vi "Configure DRAM Properties.vi"(7 "DRAM FIFO Depth":u8(ring)=20 items=["4"=2, "8"=3, "16"=4, "32"=5, "64"=6, "128"=7, "256"=8, "512"=9, "1024"=10, "2048"=11, "4096"=12, "8192"=13, "16384"=14, "32768"=15, "65536"=16, "131072"=17, "262144"=18, "524288"=19, "1048576"=20, "2097152"=21, "4194304"=22, "8388608"=23, "16777216"=24, "33554432"=25, "67108864"=26, "134217728"=27, "268435456"=28, "536870912"=29, "1073741824"=30, "2147483648"=31, "4294967296"=32], 8 "error in":errorcluster, 9 "DRAM Duty Cycle":T1={"DRAM Write Ticks"=1000, "DRAM Read Ticks"=1}, 11 "FPGA VI Reference In":refnum<k20>) -> (0 "error out":errorcluster, 3 "FPGA VI Reference Out":refnum<k20>)   [LabVIEW 2012]
uses:
  <vilib>/Utility/error.llb/Error Cluster From Error Code.vi
  <vilib>/rvi/errors/niLvFpgaAdjustHostInterfaceError.vi
  <vilib>/rvi/interface/nirviReadWriteControl/nirviReadWriteControl.xnode
  NiFpgaLv.dll
  <vilib>/rvi/interface/Simulation/niFpgaSimulationCallBeginRW.vi
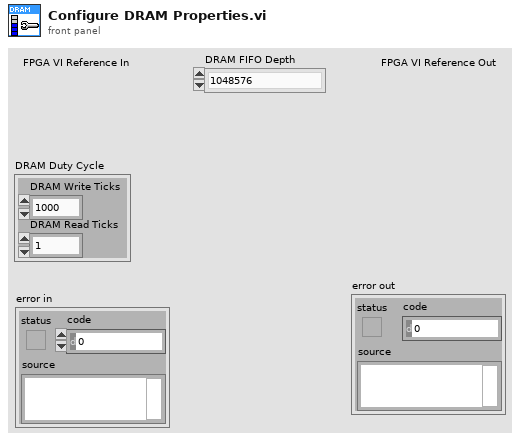
[diagram p1: front panel]
types:
  T1 = cluster{"DRAM Write Ticks":u16, "DRAM Read Ticks":u16}
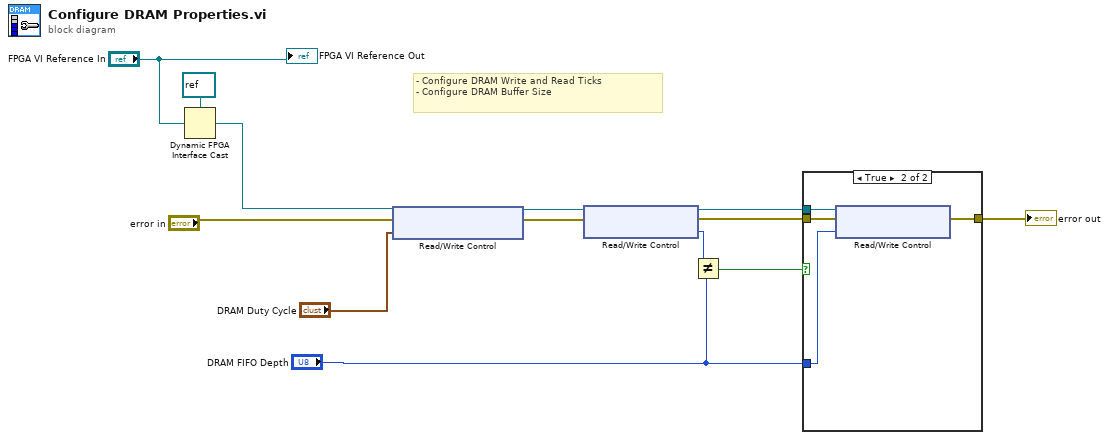
[diagram p0: block diagram]
diagram:
  # "- Configure DRAM Write and Read Ticks\n- Configure DRAM Buffer Size"
  n1 = Dynamic FPGA Interface Cast(Session In=refnum<k20> refnum ("Type"), Type="FPGA VI Reference In") -> (Session Out=w11:refnum<k20>)
  n2 = xnode "Read/Write Control"("FPGA VI Reference In"=w11, "error in"="error in", "DRAM Arbiter Config"="DRAM Duty Cycle") -> ("FPGA VI Reference Out"=w7:refnum<k20>, "error out"=w6:errorcluster)
  n3 = xnode "Read/Write Control"("FPGA VI Reference In"=w7, "error in"=w6) -> ("FPGA VI Reference Out"=w5:refnum<k20>, "error out"=w4:errorcluster, "DRAM FIFO Depth"=w3:u8)
  n4 = Not Equal?(x=w3, y="DRAM FIFO Depth") -> (x != y?=w2:bool)
  n5 = case shown="True" w2 {
    tunnel: [w14 w18] -> w8
    tunnel: w5 -> [_ w17]
    tunnel: w4 -> [w14 w16]
    tunnel: "DRAM FIFO Depth" -> [_ w15]
    frame False {
    }
    frame True {
      n6 = xnode "Read/Write Control"("FPGA VI Reference In"=w17, "error in"=w16, "DRAM FIFO Depth"=w15) -> ("error out"=w18:errorcluster)  [unwired: 1 out]
    }
  }
  "error out" <- w8
  "FPGA VI Reference Out" <- "FPGA VI Reference In"
